vi "GFITS_Gbls.vi"() -> ()   [LabVIEW 2016]
panel:
  in  "GFITS_quickhdrs":bool
  in  "GFITS_Def_Head_timing":string="after"
  out "GFITS_Headers":string[][][](array[string])
  out "GFITS_Geometry":string[][][](array[string])
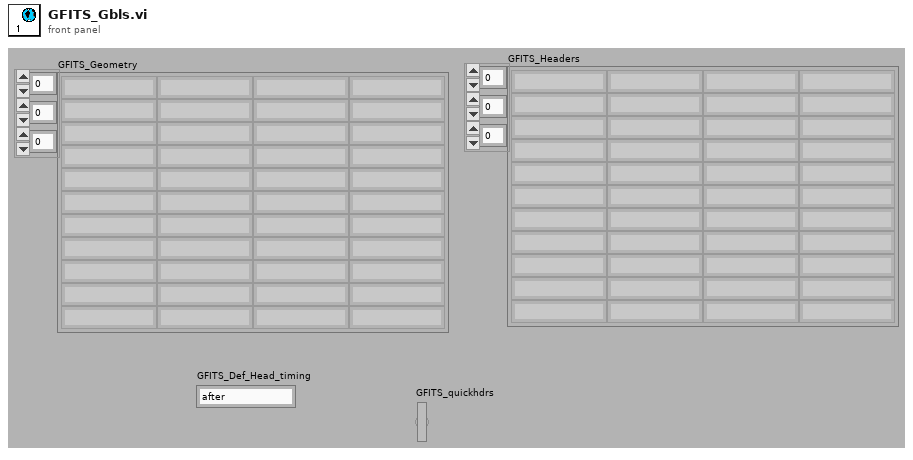
[diagram p1: front panel]
diagram:
